vi "DestroyAllUserEvents.vi"(8 "error in (no error)":errorcluster, 11 "Event Cluster":T1) -> (0 "error out":errorcluster)   [LabVIEW 2016, in "User Events.lvlib"]
uses:
  User Events.lvlib
  controls/UI Events.ctl
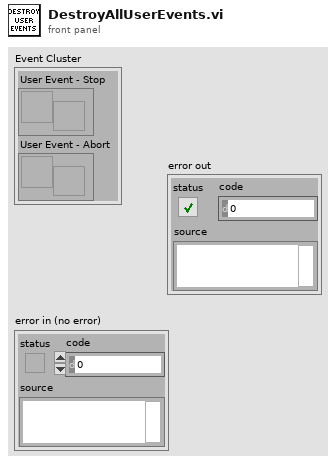
[diagram p1: front panel]
types:
  T1 = typedef "UI Events.ctl" = cluster{"User Event - Stop":refnum<user-event>, "User Event - Abort":refnum<user-event>}
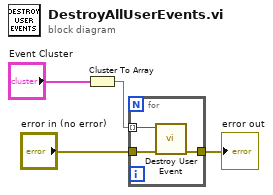
[diagram p0: block diagram]
diagram:
  n1 = Cluster To Array(cluster="Event Cluster") -> (array=w2:refnum<user-event>[])
  n2 = for {
    tunnel: [w7] -> w4
    tunnel: w2 -> [w5] mode=indexing
    tunnel: "error in (no error)" -> [w6]
    n3 = call "Destroy User Event.vi"("error in (no error)"=w6, "User Event"=w5) -> ("error out"=w7:errorcluster)  [unwired: 9 in]
  }
  "error out" <- w4
